vi "Find PeaksValleys.vi"(4 "peaks/valleys":enum32{"Peaks", "Valleys"}(ring), 6 "Options":T1, 8 "error in (no error)":errorcluster, 9 "Data Array":dbl[](array[numeric]), 10 "XYGraph in":refnum<vi>, 11 "input picture in":picture) -> (0 "error out":errorcluster, 2 "XYGraph out":refnum<vi>, 3 "input picture out":picture)   [LabVIEW 2015]
uses:
  <vilib>/Analysis/NI_AAL_SigProc.lvlib
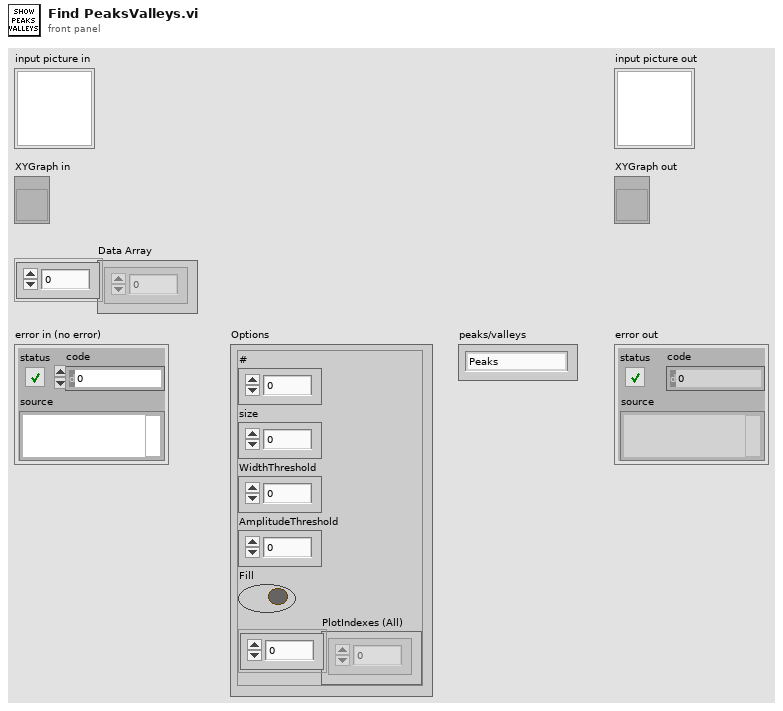
[diagram p1: front panel]
types:
  T1 = cluster{"#":i32, "size":i16, "WidthThreshold":i32, "AmplitudeThreshold":dbl, "Fill":bool, "PlotIndexes (All)":u16[]}
  T2 = typedef "LVRectTypeDef.ctl" = cluster{"Left":i16, "Top":i16, "Right":i16, "Bottom":i16}
  T3 = typedef "LVPoint32TypeDef.ctl" = cluster{"Horizontal":i32, "Vertical":i32}
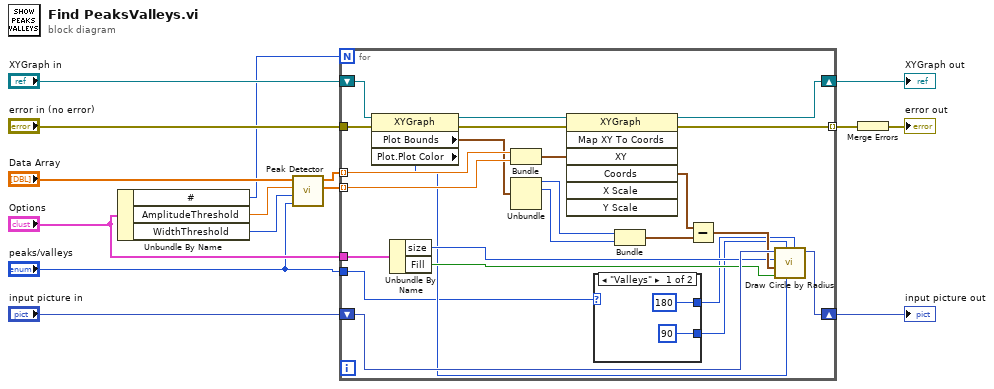
[diagram p0: block diagram]
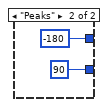
[diagram p2: hidden frame]
diagram:
  n1 = Unbundle By Name("Options") -> ("#"=w1:i32, "AmplitudeThreshold"=w14:dbl, "WidthThreshold"=w13:i32)
  n2 = call <vilib>:"Peak Detector.vi"("peaks/valleys"="peaks/valleys", "width"=w13, "threshold"=w14, "X"="Data Array") -> ("Amplitudes"=w9:dbl[], "Locations"=w8:dbl[])  [unwired: 3 in, 3 out]
  n3 = for {
    N: w1 -> [_]
    tunnel: "Options" -> [w29]
    tunnel: w8 -> [w39] mode=indexing
    tunnel: w9 -> [w38] mode=indexing
    shift-right: [w36] -> w11
    shift-left: "input picture in" -> [w37]
    shift-right: [w26] -> w4
    shift-left: "XYGraph in" -> [w25]
    tunnel: "error in (no error)" -> [w21]
    tunnel: [w19] -> w5 mode=indexing
    tunnel: "peaks/valleys" -> [w16]
    n4 = property class="XYGraph"(reference=w25, error in=w21) -> (reference out=w24:refnum<vi>, error out=w20:errorcluster, "Plot Bounds"=w22:T2, "Plot.Plot Color"=w23:u32)
    n5 = Unbundle By Name(w29) -> ("size"=w28:i16, "Fill"=w27:bool)
    n6 = Bundle(w39, w38) -> (w35:cluster{dbl, dbl})  [unwired: 1 in]
    n7 = Unbundle(w22) -> ("Left"=w33:i16, "Top"=w32:i16)  [unwired: 2 out]
    n8 = invoke on="Invoke Node" class="XYGraph" method="Map XY To Coords"(reference=w24, error in=w20, "XY"=w35) -> (reference out=w26:refnum<vi>, error out=w19:errorcluster, "Coords"=w31:T3)  [unwired: 4 in, 4 out]
    n9 = case shown="\"Valleys\"" w16 {
      tunnel: [i16 90 ("start angle(0)") i16 90 ("start angle(0)")] -> w18
      tunnel: [i16 180 ("start angle(0)") i16 -180 ("start angle(0)")] -> w17
      frame "Valleys" {
      }
      frame "Peaks" {
      }
    }
    n10 = Bundle("Left"=w33, "Top"=w32) -> (w34:cluster{"Left":i16, "Top":i16})  [unwired: 1 in]
    n11 = Subtract(x=w31, y=w34) -> (x-y=w30:T3)
    n12 = call <vilib>:"Draw Circle by Radius.vi"("arc size(360)"=w17, "color(black)"=w23, "start angle(0)"=w18, "fill?(F)"=w27, "pixel center"=w30, "radius"=w28, "picture"=w37) -> ("new picture"=w36:picture)  [unwired: 4 in]
  }
  "input picture out" <- w11
  "XYGraph out" <- w4
  n13 = Merge Errors(w5) -> (→"error out":errorcluster)
